vi "插入测量记录.vi"   [LabVIEW 2025]
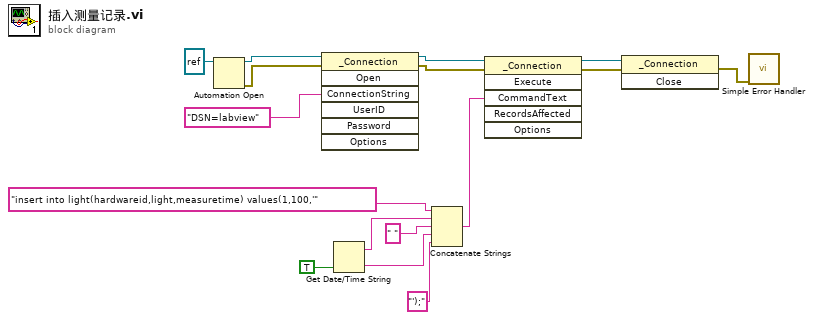
[diagram p0: block diagram]
diagram:
  n1 = Automation Open(Automation Refnum=refnum<k7> refnum ("ADODB._Connection")) -> (Automation Refnum=w2:refnum<k7>, error out=w3:errorcluster)  [unwired: 3 in]
  n2 = invoke on="调用节点" class="_Connection" method="Open"(reference=w2, error in=w3, "ConnectionString"="DSN=labview") -> (reference out=w5:refnum<k7>, error out=w4:errorcluster)  [unwired: 4 in, 5 out]
  n3 = Get Date/Time String(want seconds? (F)=TRUE) -> (date string=w13:string, time string=w11:string)  [unwired: 2 in]
  n4 = Concatenate Strings("insert into light(hardwareid,light,measuretime) values(1,100,'" ("CommandText"), w13, " " ("string"), w11, "');" ("string")) -> (w9:string)
  n5 = invoke class="_Connection" method="Execute"(reference=w5, error in=w4, "CommandText"=w9) -> (reference out=w8:refnum<k7>, error out=w7:errorcluster)  [unwired: 3 in, 4 out]
  n6 = invoke class="_Connection" method="Close"(reference=w8, error in=w7) -> (error out=w6:errorcluster)  [unwired: 1 in, 2 out]
  n7 = call <vilib>:"Simple Error Handler.vi"("error in (no error)"=w6) -> ()  [unwired: 4 in, 5 out]
